vi "Test.vi"() -> ()   [LabVIEW 2015, in "Route Manager.lvclass"]
uses:
  Route Manager.lvclass
  SLSC Switch/Controls/Path Capability.ctl
  Connection.ctl
  Position.ctl
  SLSC Switch/SLSC Switch.lvclass
panel:
  out "position":T1=10 items=["Open"=10, "Closed"=11]
  out "connections":T2[](array[typedef])
  out "error out":errorcluster
  out "relays to open 2":i32[](array[numeric])
  out "relays to close 2":i32[](array[numeric])
  out "relays to open":i32[](array[numeric])
  out "relays to close":i32[](array[numeric])
  out "path capability":T3=1 items=["Path Available"=1, "Path Exists"=2, "Path Unsupported"=3, "Resource in Use"=4, "Source Conflict"=5, "Channel Not Available"=6]
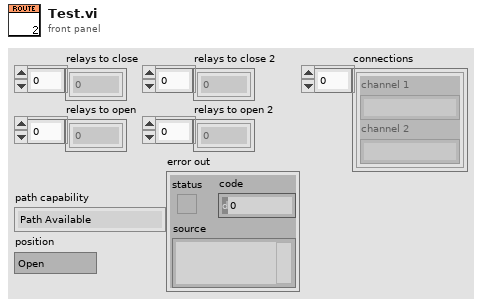
[diagram p1: front panel]
types:
  T1 = typedef "Route Manager.lvclass/Position.ctl" = i32
  T2 = typedef "Route Manager.lvclass/Connection.ctl" = cluster{"channel 1":string, "channel 2":string}
  T3 = typedef "SLSC Switch.lvclass/Path Capability.ctl" = i32
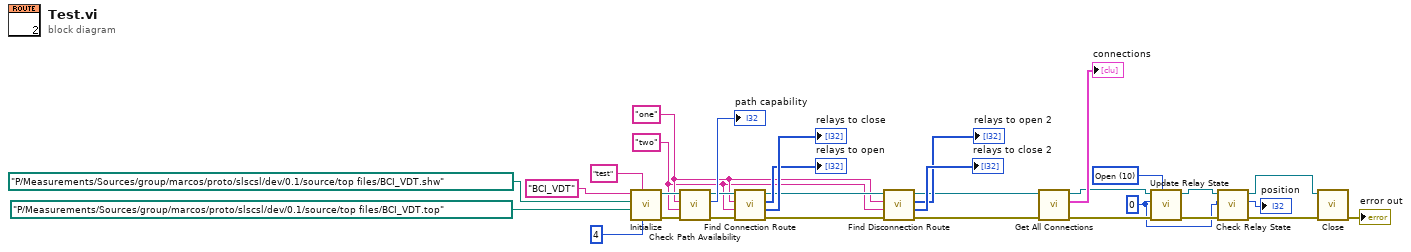
[diagram p0: block diagram]
diagram:
  w1 = 0 ("relay index")
  w8 = T1 10 items=["Open"=10, "Closed"=11] ("position")
  w17 = "two" ("channel 2")
  w18 = "one" ("channel 1")
  n1 = call "Initialize.vi"("RelayCount"=4, "deviceIdentifier"="test", "top file path"=path "P:/Measurements/Sources/group/marcos/proto/slscsl/dev/0.1/source/top files/BCI_VDT.top", "shw file path"=path "P:/Measurements/Sources/group/marcos/proto/slscsl/dev/0.1/source/top files/BCI_VDT.shw", "topologyName"="BCI_VDT") -> ("error out"=w26:errorcluster, "Route Manager out"=w27:refnum<class "Route Manager.lvclass">)  [unwired: 5 in]
  n2 = call "Check Path Availability.vi"("error in (no error)"=w26, "channel 2"=w17, "channel 1"=w18, "Route Manager in"=w27) -> ("error out"=w23:errorcluster, "path capability"=→"path capability":T3, "Route Manager out"=w24:refnum<class "Route Manager.lvclass">)  [unwired: 5 in]
  n3 = call "Find Connection Route.vi"("error in (no error)"=w23, "channel 2"=w17, "channel 1"=w18, "Route Manager in"=w24) -> ("error out"=w16:errorcluster, "relays to close"=→"relays to close":i32[], "relays to open"=→"relays to open":i32[], "Route Manager out"=w19:refnum<class "Route Manager.lvclass">)  [unwired: 4 in]
  n4 = call "Find Disconnection Route.vi"("error in (no error)"=w16, "channel 2"=w17, "channel 1"=w18, "Route Manager in"=w19) -> ("error out"=w11:errorcluster, "relays to close"=→"relays to close 2":i32[], "relays to open"=→"relays to open 2":i32[], "Route Manager out"=w12:refnum<class "Route Manager.lvclass">)  [unwired: 4 in]
  n5 = call "Get All Connections.vi"("error in (no error)"=w11, "Route Manager in"=w12) -> ("error out"=w7:errorcluster, "connections"=→"connections":T2[], "Route Manager out"=w4:refnum<class "Route Manager.lvclass">)  [unwired: 7 in]
  n6 = call "Update Relay State.vi"("position"=w8, "error in (no error)"=w7, "relay index"=w1, "Route Manager in"=w4) -> ("error out"=w6:errorcluster, "Route Manager out"=w3:refnum<class "Route Manager.lvclass">)  [unwired: 6 in]
  n7 = call "Check Relay State.vi"("error in (no error)"=w6, "relay index"=w1, "Route Manager in"=w3) -> ("error out"=w5:errorcluster, "position"=→"position":T1, "Route Manager out"=w2:refnum<class "Route Manager.lvclass">)  [unwired: 6 in]
  n8 = call "Close.vi"("error in (no error)"=w5, "Route Manager in"=w2) -> ("error out"=→"error out":errorcluster)  [unwired: 9 in]
